vi "Ridders Zero Finder (Formula).vi"(8 "formula":string, 9 "end":dbl=1.0 format="%.2f", 10 "start":dbl format="%.2f", 11 "accuracy":dbl=1e-08 format="%.2e") -> (0 "error":i32, 1 "ticks":u32, 2 "f(zero)":dbl format="%.2f", 3 "zero":dbl format="%.2f")   [LabVIEW 2017, in "NI_Gmath.lvlib"]
doc: "Determines a zero of a 1D function in a given interval. The function has to be continuous and has to have different signs at the end points of the interval. You must manually select the polymorphic instance to use."
uses:
  NI_Gmath.lvlib
panel:
  # "Example:\n\n accuracy: 1E-8 \n start: 0.0\n end: 1.0\n formula: x^2+sin(x)-1"
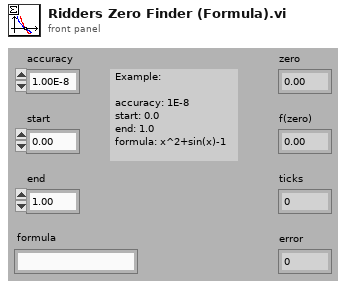
[diagram p1: front panel]
types:
  T1 = cluster{"y value":dbl, "y value":dbl, "start":dbl, "end":dbl}
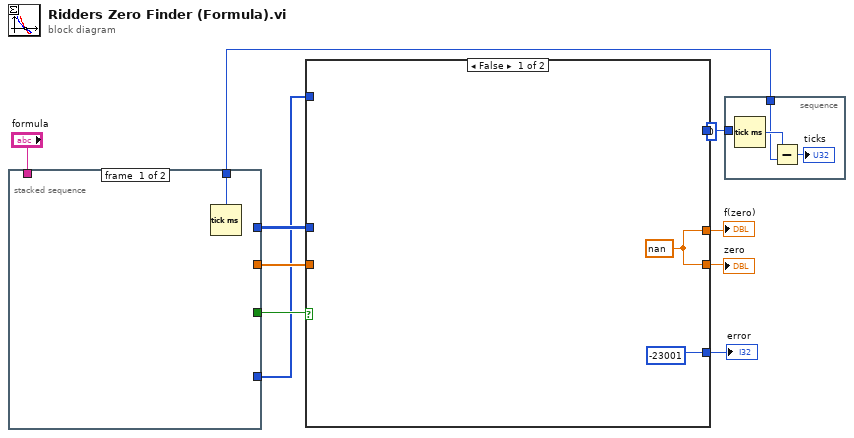
[diagram p0: block diagram]
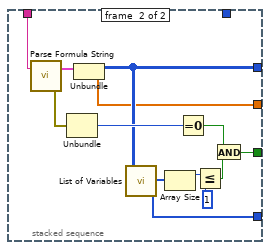
[diagram p2: hidden frame]
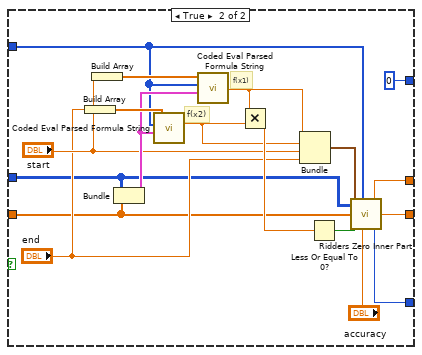
[diagram p3: hidden frame]
diagram:
  n1 = stacked-sequence {
    tunnel: [_ w23] -> w10
    tunnel: [w11 _] -> w8
    tunnel: "formula" -> [_ w17]
    tunnel: [_ w13] -> w3
    tunnel: [_ w12] -> w2
    tunnel: [_ w18] -> w1
    frame #0 {
      n2 = Tick Count (ms)() -> (millisecond timer value=w11:u32)
    }
    frame #1 {
      n3 = call "Parse Formula String.vi"("formula"=w17) -> ("error out"=w16:errorcluster, "Parsed Formula"=w14:cluster{"Table":i32[][], "Y Values":dbl[]})  [unwired: 1 in]
      n4 = Unbundle(w16) -> ("code"=w15:i32)  [unwired: 2 out]
      n5 = Unbundle(w14) -> ("Table"=w13:i32[][], "Y Values"=w12:dbl[])
      n6 = call "List of Variables.vi"("Table"=w13) -> ("List of variables"=w18:i32[])
      n7 = Array Size(array=w18) -> (size(s)=w19:i32)
      n8 = Equal To 0?(x=w15) -> (x = 0?=w22:bool)
      n9 = Less Or Equal?(x=w19, y=1) -> (x <= y?=w21:bool)
      n10 = And(x=w22, y=w21) -> (x .and. y?=w23:bool)
    }
  }
  n11 = case shown="False" w10 {
    tunnel: [0 0] -> w9
    tunnel: [-23001 w41] -> w6
    tunnel: [w24 w39] -> w5
    tunnel: [w24 w38] -> w4
    tunnel: w3 -> [_ w29]
    tunnel: w2 -> [_ w28]
    tunnel: w1 -> [_ w27]
    frame False {
      w24 = nan
    }
    frame True {
      # "f(x1)"
      # "f(x2)"
      n12 = Build Array("end") -> (w36:dbl[])
      n13 = Build Array("start") -> (w37:dbl[])
      n14 = Bundle("Table"=w29, "Y Values"=w28) -> (w35:cluster{"Table":i32[][], "Y Values":dbl[]})  [unwired: 1 out]
      n15 = call "Coded Eval Parsed Formula String.vi"("Parsed Formula"=w35, "Variables"=w27, "X Values"=w36) -> ("y value"=w33:dbl)  [unwired: 1 in, 1 out]
      n16 = call "Coded Eval Parsed Formula String.vi"("Parsed Formula"=w35, "Variables"=w27, "X Values"=w37) -> ("y value"=w34:dbl)  [unwired: 1 in, 1 out]
      n17 = Multiply(x=w34, y=w33) -> (x*y=w44:dbl)
      n18 = Bundle("y value"=w34, "y value"=w33, "start"="start", "end"="end") -> (w32:T1)  [unwired: 1 out]
      n19 = Less Or Equal To 0?(x=w44) -> (x <= 0?=w43:bool)
      n20 = call "Ridders Zero Inner Part.vi"("start/end/f(x)"=w32, "list of variables"=w27, "table"=w29, "result"=w28, "accuracy"="accuracy", "case"=w43) -> ("y value"=w38:dbl, "end"=w39:dbl, "error"=w41:i32)
    }
  }
  "error" <- w6
  "zero" <- w5
  "f(zero)" <- w4
  n21 = stacked-sequence {
    tunnel: w9 -> [_]
    tunnel: w8 -> [w45]
    frame #0 {
      n22 = Tick Count (ms)() -> (millisecond timer value=w46:u32)
      n23 = Subtract(x=w46, y=w45) -> (x-y=→"ticks":u32)
    }
  }
